vi "Init.vi"(7 "Lumberjack.lvlib:Layout.lvclass":refnum<class "Layout.lvclass">, 8 "error in (no error)":errorcluster, 10 "common":T1={"id"="", "threshold"=enum."INFO", "filter"={"mode"=enum."Mirror", "levelMin"=enum."INFO", "levelMax"=enum."INFO", "tagPrefix"=""}, "queueBound"=-1, "dropPolicy"=enum."DropOldest", "useUTC"=FALSE}, 11 "ConsoleAppender in":refnum<class "ConsoleAppender.lvclass">) -> (0 "error out":errorcluster, 3 "ConsoleAppender out":refnum<class "ConsoleAppender.lvclass">)   [LabVIEW 2026, in "Lumberjack.lvlib" / "ConsoleAppender.lvclass"]
doc: "Construct a ConsoleAppender: set its layout (default TextLayout if none injected), then call InitCommon to set the common appender fields. Public creation entry point (SRS-LMBR-031)."
uses:
  ConsoleAppender.lvclass
  TypeDefs/AppenderConfig.ctl
  TypeDefs/Severity.ctl
  TypeDefs/Filter.ctl
  TypeDefs/FilterMode.ctl
  TypeDefs/DropPolicy.ctl
  Layouts/Layout.lvclass/Layout.lvclass
  ConsoleAppender.lvclass/ConsoleAppender.ctl
  Layouts/Layout.lvclass/Write useUTC.vi
  Appender.lvclass/Appender.lvclass
  Lumberjack.lvlib
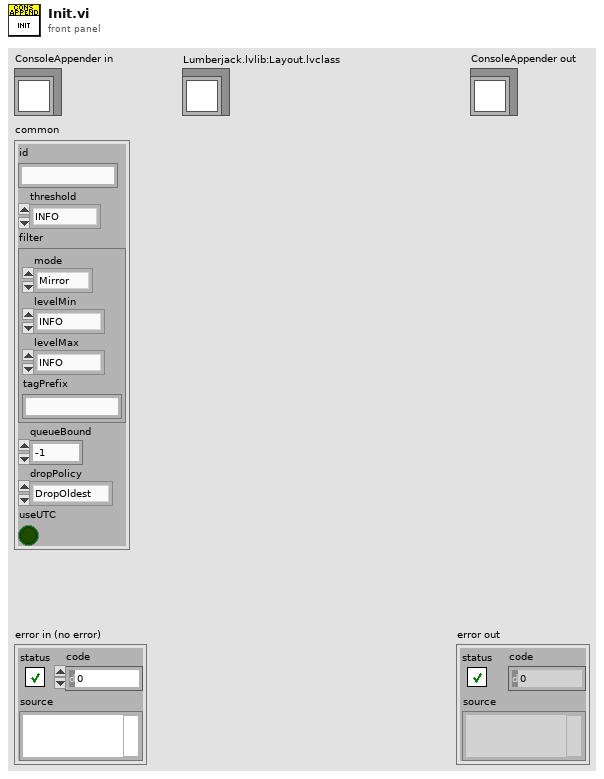
[diagram p1: front panel]
types:
  T1 = typedef "Lumberjack.lvlib/AppenderConfig.ctl" = cluster{"id":string, "threshold":T2, "filter":T3, "queueBound":i32, "dropPolicy":T5, "useUTC":bool}
  T2 = typedef "Lumberjack.lvlib/Severity.ctl" = enum16{"OFF", "FATAL", "ERROR", "WARN", "INFO", "DEBUG", "TRACE", "ALL"}
  T3 = typedef "Lumberjack.lvlib/Filter.ctl" = cluster{"mode":T4, "levelMin":T2, "levelMax":T2, "tagPrefix":string}
  T4 = typedef "Lumberjack.lvlib/FilterMode.ctl" = enum16{"Mirror", "Routed"}
  T5 = typedef "Lumberjack.lvlib/DropPolicy.ctl" = enum16{"DropOldest", "DropNewest", "LevelAware"}
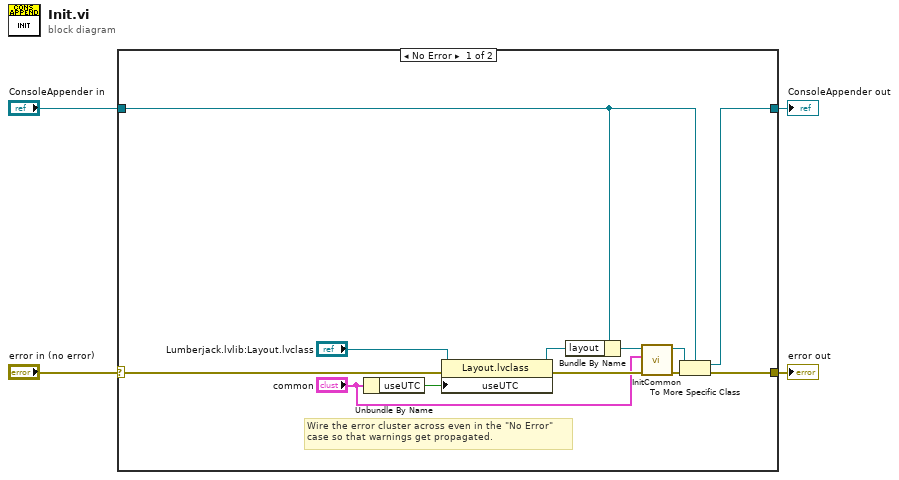
[diagram p0: block diagram]
diagram:
  n1 = case shown="No Error" "error in (no error)" {
    selector: "error in (no error)" -> [w15 w18]
    tunnel: [w8 w18] -> w3
    tunnel: [w7 w17] -> w1
    tunnel: "ConsoleAppender in" -> [w6 w17]
    frame No Error {
      # "Wire the error cluster across even in the \"No Error\"\ncase so that warnings get propagated."
      n2 = Unbundle By Name("common") -> ("useUTC"=w11:bool)
      n3 = property class="Layout.lvclass"(reference="Lumberjack.lvlib:Layout.lvclass", error in=w15, "useUTC"=w11) -> (reference out=w14:refnum<class "Layout.lvclass">, error out=w13:errorcluster)
      n4 = Bundle By Name(cluster=w6, "layout"=w14) -> (w16:refnum<class "ConsoleAppender.lvclass">)
      n5 = call "InitCommon.vi"("error in (no error)"=w13, "AppenderConfig"="common", "Appender in"=w16) -> ("error out"=w9:errorcluster, "Appender out"=w5:refnum<class "ConsoleAppender.lvclass">)  [unwired: 7 in]
      n6 = To More Specific Class(target class=w6, reference=w5, error in=w9) -> (specific class reference=w7:refnum<class "ConsoleAppender.lvclass">, error out=w8:errorcluster)
    }
    frame Error {
    }
  }
  "error out" <- w3
  "ConsoleAppender out" <- w1
